vi "Layer2_BuildTxString.vi"(1 "Message":string="TestStation1", 2 "PacketNum":i32, 3 "Control":i32=56) -> (0 "Write Buffer":string)   [LabVIEW 2012]
uses:
  Arduino_Serial_GlobalConstants.vi
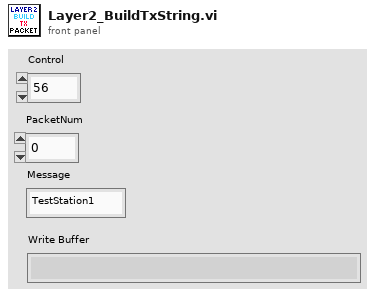
[diagram p1: front panel]
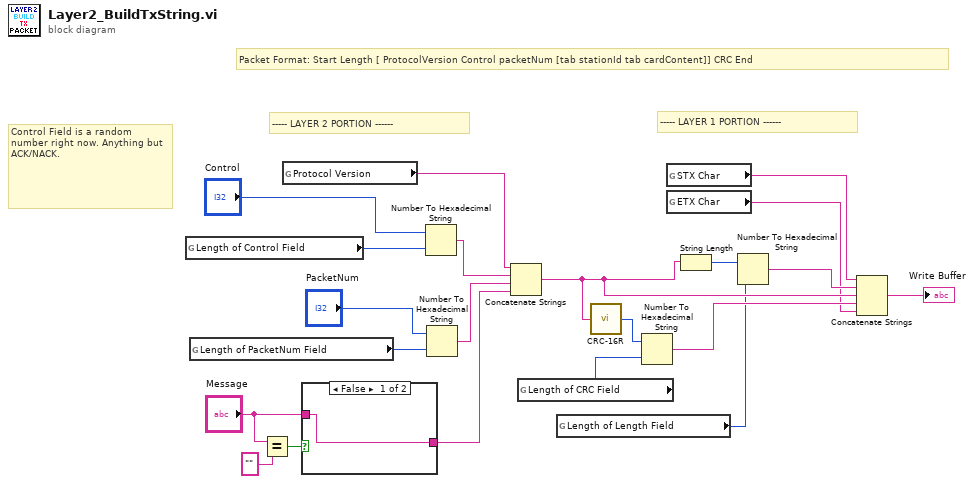
[diagram p0: block diagram]
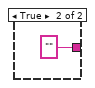
[diagram p2: hidden frame]
diagram:
  # "----- LAYER 1 PORTION ------"
  # "----- LAYER 2 PORTION ------"
  # "Control Field is a random number right now. Anything but ACK/NACK."
  # "Packet Format: Start Length [ ProtocolVersion Control packetNum [tab stationId tab cardContent]] CRC End"
  n1 = global read "Arduino_Serial_GlobalConstants.vi" "Length of Control Field"() -> (w6:i32)
  n2 = global read "Arduino_Serial_GlobalConstants.vi" "Length of PacketNum Field"() -> (w5:i32)
  n3 = Equal?(x="Message", y="") -> (x = y?=w13:bool)
  n4 = global read "Arduino_Serial_GlobalConstants.vi" "Protocol Version"() -> (w2:string)
  n5 = case shown="False" w13 {
    tunnel: [w22 "" ("y")] -> w10
    tunnel: "Message" -> [w22 _]
    frame False {
    }
    frame True {
    }
  }
  n6 = Number To Hexadecimal String(1:w6, 2:"Control") -> (0:w1:string)
  n7 = Number To Hexadecimal String(1:w5, 2:"PacketNum") -> (0:w20:string)
  n8 = Concatenate Strings(w2, w1, w20, w10) -> (w15:string)
  n9 = global read "Arduino_Serial_GlobalConstants.vi" "Length of CRC Field"() -> (w3:i32)
  n10 = global read "Arduino_Serial_GlobalConstants.vi" "Length of Length Field"() -> (w4:i32)
  n11 = call <instrlib>:"CRC-16R.vi"("String"=w15) -> ("Checksum"=w17:u16)  [unwired: 2 out]
  n12 = Number To Hexadecimal String(1:w3, 2:w17) -> (0:w16:string)
  n13 = global read "Arduino_Serial_GlobalConstants.vi" "STX Char"() -> (w8:string)
  n14 = global read "Arduino_Serial_GlobalConstants.vi" "ETX Char"() -> (w7:string)
  n15 = String Length(string=w15) -> (length=w19:i32)
  n16 = Number To Hexadecimal String(1:w4, 2:w19) -> (0:w18:string)
  n17 = Concatenate Strings(w8, w18, w15, w16, w7) -> (→"Write Buffer":string)
